vi "Go Home.vi"() -> ()   [LabVIEW 2017]
uses:
  Go Home State type def.ctl
panel:
  out "X Velocity (mm/s)":dbl format="%#_3g"
  out "Y Velocity (mm/s)":dbl format="%#_3g"
  out "Enum":T1
  out "X-axis distance":dbl
  out "Y-axis distance":dbl
  in  "stop":bool
  out "Motor Status":cluster{"Homing Freq":dbl, "Homing Duty %":dbl} {"Homing Duty %" format="%#_13g"; "Homing Freq" format="%#_13g"}
  in  "Homing Duty %":dbl format="%#_13g"
  in  "Homing Freq":dbl format="%#_13g"
  in  "error in (no error)":errorcluster
  out "error out":errorcluster
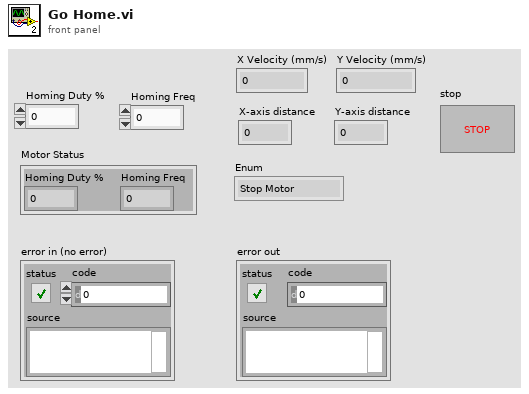
[diagram p1: front panel]
types:
  T1 = typedef "Go Home State type def.ctl" = enum16{"Stop Motor", "Read Input", "Drive Y", "Drive X"}
  T2 = typedef "Encoder Cluster.ctl" = cluster{"Y-axis rev count":dbl, "Y-axis distance":dbl, "X-axis rev count":dbl, "X-axis distance":dbl, "Y-axis direction":T3, "X-axis direction":T3, "X-counter val":i32, "Y-counter val":i32}
  T3 = typedef "Encoder Count Direction Enum.ctl" = enum16{"Counting Up", "Counting Down"}
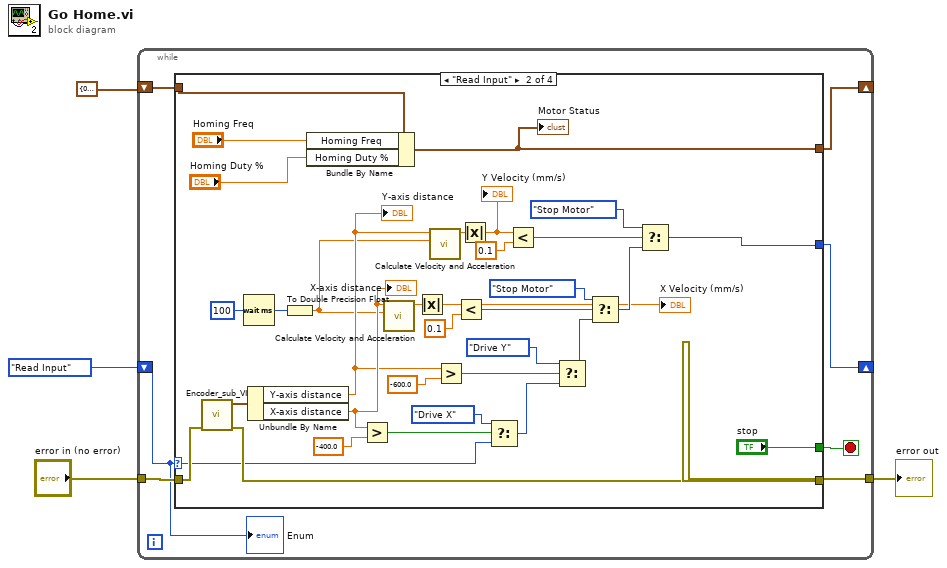
[diagram p0: block diagram]
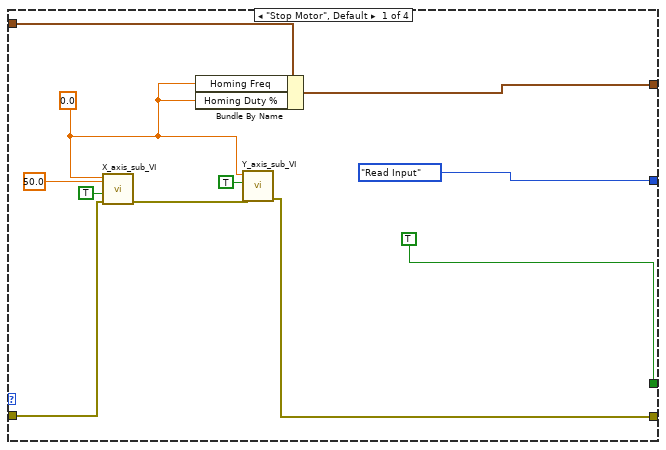
[diagram p2: hidden frame]
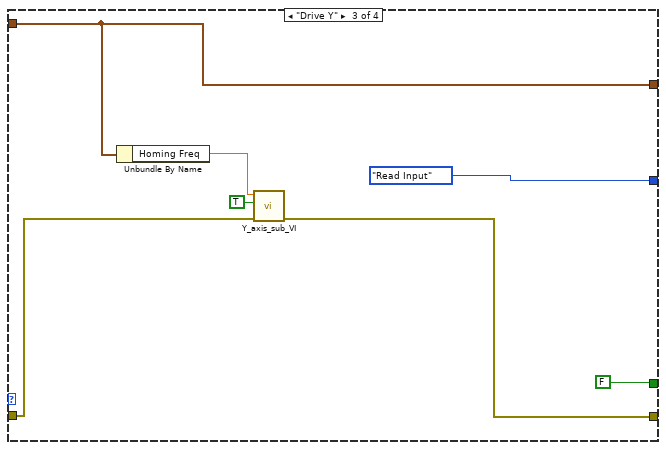
[diagram p3: hidden frame]
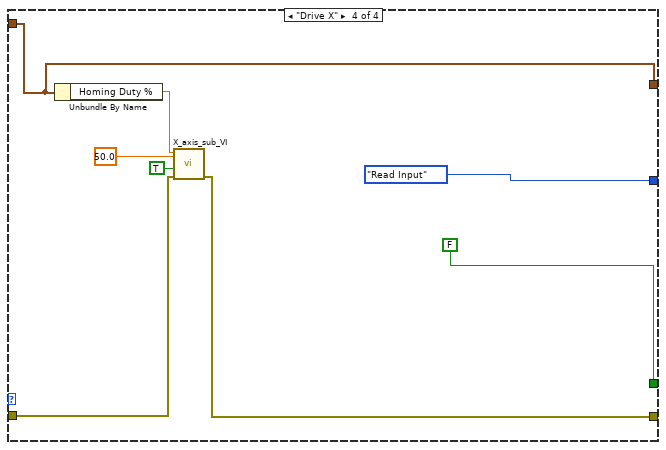
[diagram p4: hidden frame]
diagram:
  n1 = while {
    tunnel: "error in (no error)" -> [w8]
    tunnel: [w7] -> w3
    shift-right: [w9] -> _
    shift-left: Go_Home_State_type_def."Read Input" -> [w5]
    shift-right: [w10] -> _
    shift-left: cluster{"Homing Freq":dbl, "Homing Duty %":dbl} {"Homing Freq"=0.0, "Homing Duty %"=0.0} ("Cluster 2") -> [w11]
    stop <- w6 stop-if-true
    n2 = case shown="\"Read Input\"" w5 {
      selector: w5 -> [_ w40 _ _]
      tunnel: w11 -> [w22 w55 w57 w66]
      tunnel: [w21 w53 w57 w66] -> w10
      tunnel: [Go_Home_State_type_def."Read Input" w27 Go_Home_State_type_def."Read Input" Go_Home_State_type_def."Read Input"] -> w9
      tunnel: w8 -> [w18 w48 w61 w69]
      tunnel: [w19 w47 w60 w68] -> w7
      tunnel: [TRUE "stop" FALSE ("stop") FALSE ("stop")] -> w6
      frame "Stop Motor", Default {
        w17 = 0.0
        n3 = call "X_axis_sub_VI.vi"("error in (no error)"=w18, "FWD/RVS"=TRUE, "Frequency"=50.0, "Duty Cycle %"=w17) -> ("error out"=w20:errorcluster)  [unwired: 7 in]
        n4 = Bundle By Name(cluster=w22, "Homing Freq"=w17, "Homing Duty %"=w17) -> (w21:cluster{"Homing Freq":dbl, "Homing Duty %":dbl})
        n5 = call "Y_axis_sub_VI.vi"("error in (no error)"=w20, "FWD/RVS"=TRUE, "Frequency"=w17) -> ("error out"=w19:errorcluster)  [unwired: 8 in]
      }
      frame "Read Input" {
        n6 = call "Encoder_sub_VI.vi"("error in (no error)"=w48) -> ("error out"=w47:errorcluster, "Encoder Output"=w52:T2)  [unwired: 9 in]
        n7 = Wait (ms)(milliseconds to wait=u32 100) -> (millisecond timer value=w39:u32)
        n8 = Unbundle By Name(w52) -> ("Y-axis distance"=w33:dbl, "X-axis distance"=w38:dbl)
        "Y-axis distance" <- w33
        "X-axis distance" <- w38
        n9 = To Double Precision Float(number=w39) -> (double precision float=w32:dbl)
        n10 = Bundle By Name(cluster=w55, "Homing Freq"="Homing Freq", "Homing Duty %"="Homing Duty %") -> (w53:cluster{"Homing Freq":dbl, "Homing Duty %":dbl})
        "Motor Status" <- w53
        n11 = Greater?(x=w38, y=-400.0) -> (0:w43:bool)
        n12 = call "Calculate Velocity and Acceleration.vi"("Loop Runtime (s)"=w32, "Displacement (mm)"=w38) -> ("Velocity (mm/s)"=w37:dbl)  [unwired: 8 in, 1 out]
        n13 = Absolute Value(x=w37) -> (abs(x)=w23:dbl)
        "X Velocity (mm/s)" <- w23
        n14 = call "Calculate Velocity and Acceleration.vi"("Loop Runtime (s)"=w32, "Displacement (mm)"=w33) -> ("Velocity (mm/s)"=w30:dbl)  [unwired: 8 in, 1 out]
        n15 = Greater?(x=w33, y=-600.0) -> (0:w41:bool)
        n16 = Less?(x=w23, y=0.1) -> (x < y?=w35:bool)
        n17 = Absolute Value(x=w30) -> (abs(x)=w24:dbl)
        "Y Velocity (mm/s)" <- w24
        n18 = Select(t=Go_Home_State_type_def."Drive X", s=w43, f=w40) -> (s? t:f=w50:T1)
        n19 = Less?(x=w24, y=0.1) -> (x < y?=w29:bool)
        n20 = Select(t=Go_Home_State_type_def."Drive Y", s=w41, f=w50) -> (s? t:f=w34:T1)
        n21 = Select(t=Go_Home_State_type_def."Stop Motor", s=w35, f=w34) -> (s? t:f=w28:T1)
        n22 = Select(t=Go_Home_State_type_def."Stop Motor", s=w29, f=w28) -> (s? t:f=w27:T1)
      }
      frame "Drive Y" {
        n23 = Unbundle By Name(w57) -> ("Homing Freq"=w58:dbl)
        n24 = call "Y_axis_sub_VI.vi"("error in (no error)"=w61, "FWD/RVS"=TRUE, "Frequency"=w58) -> ("error out"=w60:errorcluster)  [unwired: 8 in]
      }
      frame "Drive X" {
        n25 = Unbundle By Name(w66) -> ("Homing Duty %"=w67:dbl)
        n26 = call "X_axis_sub_VI.vi"("error in (no error)"=w69, "FWD/RVS"=TRUE, "Frequency"=50.0, "Duty Cycle %"=w67) -> ("error out"=w68:errorcluster)  [unwired: 7 in]
      }
    }
    "Enum" <- w5
  }
  "error out" <- w3
